vi "LSX Get Joystick.vi"(0 "lLSID":i32, 1 "pbEncoder":i32, 5 "pbJoystickOn":i32, 7 "pbManual":i32, 9 "pbPositionCount":i32, 11 "error in (no error)":errorcluster) -> (3 "pbEncoder out":i32, 4 "function return":i32, 6 "pbJoystickOn out":i32, 8 "pbManual out":i32, 10 "pbPositionCount out":i32, 15 "error out":errorcluster)   [LabVIEW 2018, in "Tango.lvlib"]
doc: "TANGOAPI int TANGOCALL LSX_GetJoystick (int lLSID, BOOL *pbJoystickOn, BOOL *pbManual, BOOL *pbPositionCount, BOOL *pbEncoder);"
uses:
  Tango.lvlib
  SubVIs/Tango_DLL.dll
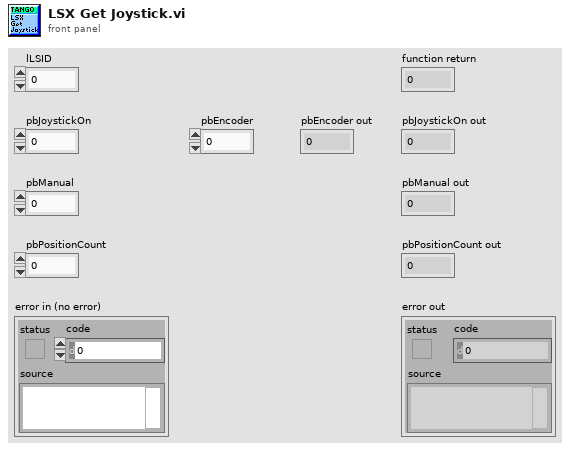
[diagram p1: front panel]
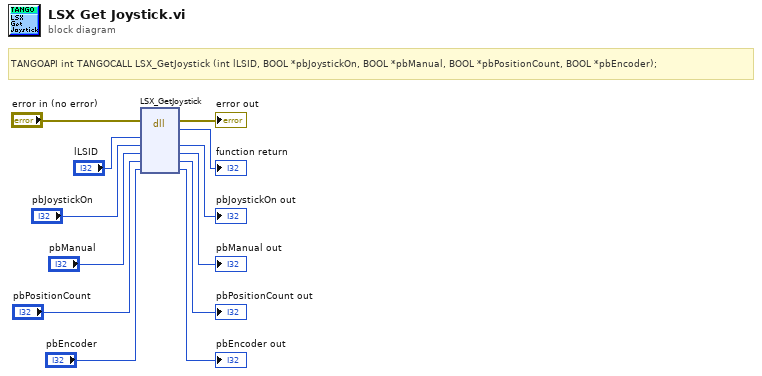
[diagram p0: block diagram]
diagram:
  # "TANGOAPI int TANGOCALL LSX_GetJoystick (int lLSID, BOOL *pbJoystickOn, BOOL *pbManual, BOOL *pbPositionCount, BOOL *pbEncoder);"
  n1 = dll-call lib="C:/Users/Familie/Documents/LabviewIX81/lib/TANGO Stage/SubVIs/Tango_DLL.*" fn="LSX_GetJoystick"(error in="error in (no error)", "lLSID"="lLSID", "pbJoystickOn"="pbJoystickOn", "pbManual"="pbManual", "pbPositionCount"="pbPositionCount", "pbEncoder"="pbEncoder") -> (error out=→"error out":errorcluster, →"function return":i32, "pbJoystickOn"=→"pbJoystickOn out":i32, "pbManual"=→"pbManual out":i32, "pbPositionCount"=→"pbPositionCount out":i32, "pbEncoder"=→"pbEncoder out":i32)  [unwired: 3 in, 1 out]
